vi "Set CompactSubObj.vi"(8 "error in":errorcluster, 10 "Value":refnum<class "Value.lvclass">, 11 "DOMAIN in":refnum<class "DOMAIN.lvclass">) -> (0 "error out":errorcluster, 3 "DOMAIN out":refnum<class "DOMAIN.lvclass">)   [LabVIEW 2024, in "Electronic Datasheet.lvlib" / "DOMAIN.lvclass"]
uses:
  DOMAIN.lvclass
  DOMAIN.lvclass/DOMAIN.ctl
  Value/Value.lvclass
  Electronic Datasheet.lvlib
  D:/git/EDS-File-Viewer/Core/Object Type/Object Type Base.lvclass
  D:/git/EDS-File-Viewer/Core/DOMAIN/DOMAIN.lvclass
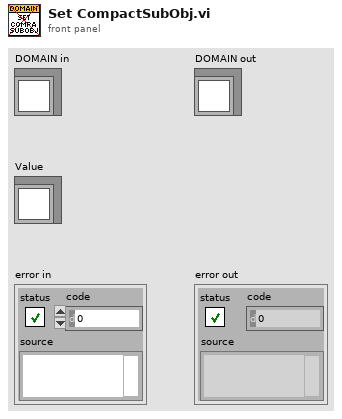
[diagram p1: front panel]
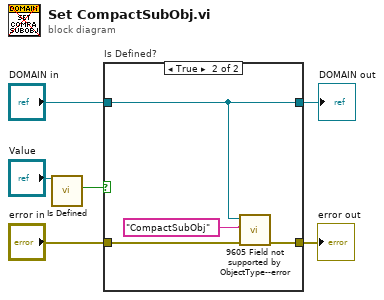
[diagram p0: block diagram]
diagram:
  n1 = call "Is Defined.vi"("Value in"="Value") -> ("Is Defined?"=w5:bool)  [unwired: 9 in, 1 out]
  n2 = case "Is Defined?" shown="True" w5 {
    tunnel: "error in" -> [w8 w12]
    tunnel: "DOMAIN in" -> [w7 w9]
    tunnel: [w8 w11] -> w2
    tunnel: [w7 w9] -> w1
    frame False {
    }
    frame True {
      n3 = call "9605 Field not supported by ObjectType--error.vi"("error in"=w12, "Field Name"="CompactSubObj" ("Field name"), "Object Type Base"=w9) -> ("error out"=w11:errorcluster)  [unwired: 8 in]
    }
  }
  "error out" <- w2
  "DOMAIN out" <- w1
